vi "Read DImodified.vi"(8 "error in (no error)":errorcluster, 11 "DI in":T1) -> (0 "error out":errorcluster, 2 "modified":u8, 3 "DI out":T1)   [LabVIEW 2019, in "Inputs.lvlib"]
uses:
  Inputs.lvlib
  Ctl/DI.ctl
  Ctl/DI short.ctl
  Ctl/Parameter State.ctl
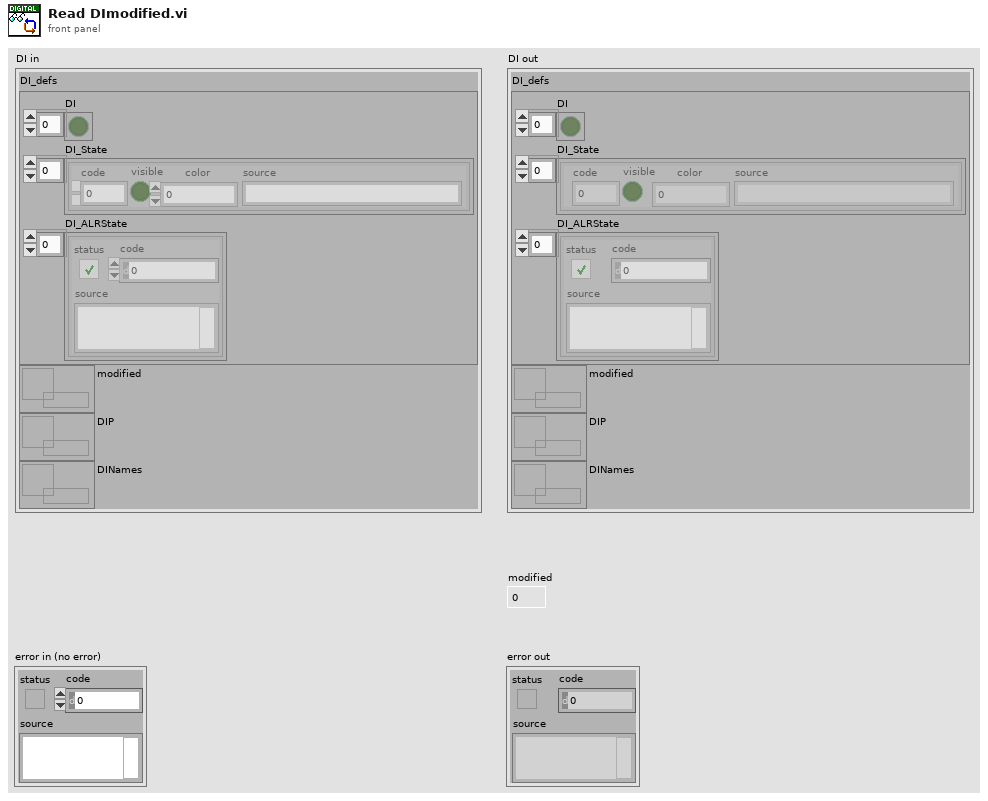
[diagram p1: front panel]
types:
  T1 = typedef "Inputs.lvlib/DI.ctl" = cluster{"DI_defs":T2, "modified":refnum<data-value>, "DIP":refnum<data-value>, "DINames":refnum<data-value>}
  T2 = typedef "Inputs.lvlib/DI short.ctl" = cluster{"DI":bool[], "DI_State":T3[], "DI_ALRState":errorcluster[]}
  T3 = typedef "Inputs.lvlib/Parameter State.ctl" = cluster{"code":i32, "visible":bool, "color":u32, "source":string}
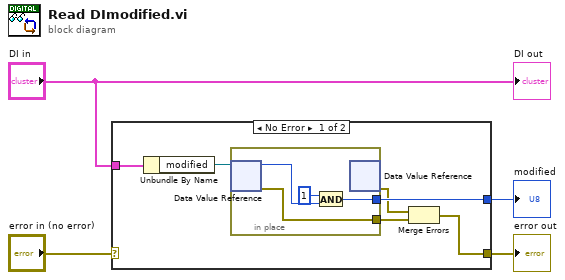
[diagram p0: block diagram]
diagram:
  n1 = case shown="No Error" "error in (no error)" {
    selector: "error in (no error)" -> [_ w15]
    tunnel: [w6 w15] -> w1
    tunnel: "DI in" -> [w5 _]
    tunnel: [w9 _] -> w2
    frame No Error {
      n2 = Unbundle By Name(w5) -> ("modified"=w10:refnum<data-value>)
      n3 = in-place {
        in-place-border: [w14] -> w8
        in-place-border: [w12] -> w9
        n4 = in-place-dvr #1(w10) -> (w13:u8, w14:errorcluster)
        n5 = And(x=u8 1, y=w13) -> (x .and. y?=w12:u8)
        n6 = in-place-dvr #1() -> (w7:errorcluster)  [unwired: 1 in, 1 out]
      }
      n7 = Merge Errors(w7, w8) -> (w6:errorcluster)
    }
    frame Error {
    }
  }
  "error out" <- w1
  "modified" <- w2
  "DI out" <- "DI in"
